vi "Get DDGIOC Trigger.vi"(8 "error in (no error)":errorcluster, 11 "trigger":u32) -> (0 "error out":errorcluster, 2 "function return":u32, 3 "trigger out":u32)   [LabVIEW 2014, in "atmcd32d.lvlib"]
doc: "unsigned int WINAPI GetDDGIOCTrigger(at_u32 * trigger);"
uses:
  atmcd32d.lvlib
  atmcd32d.dll
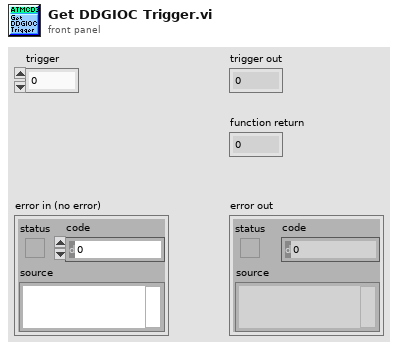
[diagram p1: front panel]
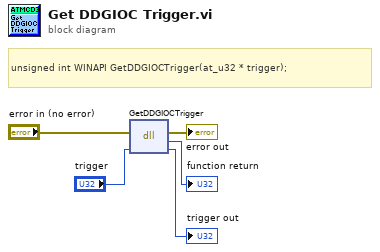
[diagram p0: block diagram]
diagram:
  # "unsigned int WINAPI GetDDGIOCTrigger(at_u32 * trigger);"
  n1 = dll-call lib="C:/Users/Bakir/Documents/Lambda2-Testing/lib/Andorlib/atmcd32d.*" fn="GetDDGIOCTrigger"(error in="error in (no error)", "trigger"="trigger") -> (error out=→"error out":errorcluster, →"function return":u32, "trigger"=→"trigger out":u32)  [unwired: 2 in, 1 out]
